vi "S4GUI.vi"(7 "Tab ObsEng":enum32{"Obs", "CCD modes", "Eng"}(tab)) -> ()   [LabVIEW 2018] (continued)
            n3853 = call-dynamic "Write sequencia.vi"("error in (no error)"=w8967, "sequencia"=w8969, "Opt_Selector in"=w8970) -> ("error out"=w8962:errorcluster, "Opt_Selector out"=w8963:refnum<class "Opt_Selector.lvclass">)  [unwired: 7 in]
            n3854 = call-dynamic "Read State Machine.vi"("error in (no error)"=w8962, "Device in"=w8963) -> ("error out"=w8965:errorcluster, "State Machine.lvclass"=w8960:refnum<class "State Machine.lvclass">, "Device out"=w8961:refnum<class "Opt_Selector.lvclass">)  [unwired: 7 in]
            n3855 = call "Next State.vi"("error in (no error)"=w8965, "New_State"=10, "State Machine in"=w8960) -> ("error out"=w8964:errorcluster, "State Machine out"=w8959:refnum<class "State Machine.lvclass">)  [unwired: 7 in]
            n3856 = call-dynamic "Write State Machine.vi"("error in (no error)"=w8964, "State Machine.lvclass"=w8959, "Device in"=w8961) -> ("error out"=w8958:errorcluster, "Device out"=w8957:refnum<class "Opt_Selector.lvclass">)  [unwired: 7 in]
            n3857 = call "Write WPROT.vi"("error in (no error)"=w8958, "Opt_Selector.lvclass"=w8957, "Instrument in"=w8976) -> ("error out"=w8955:errorcluster, "Instrument out"=w8956:refnum<class "Instrument.lvclass">)  [unwired: 7 in]
            n3858 = call "Write Instrument.lvclass.vi"("error in (no error)"=w8955, "Instrument.lvclass"=w8956, "S4ACS_GUI in"=w8974) -> ("error out"=w8977:errorcluster, "S4ACS_GUI out"=w8978:refnum<class "S4GUI.lvclass">)  [unwired: 7 in]
            n3859 = call-dynamic "Write ciclos.vi"("error in (no error)"=w8977, "ciclos"=u32 0, "S4ACS_GUI in"=w8978) -> ("error out"=w8951:errorcluster, "S4ACS_GUI out"=w8952:refnum<class "S4GUI.lvclass">)  [unwired: 7 in]
          }
          frame Enabled {
            w9068 = FALSE ("Wait Until Done")
            n3860 = call <vilib>:"Application Directory.vi"() -> ("Application Directory"=w9063:path)
            n3861 = Build Path(base path=w9063, name or relative path="MsgAbortSync.vi") -> (appended path=w9071:path)
            n3862 = Open VI Reference(vi path=w9071, error in (no error)=w9066) -> (vi reference=w9070:refnum<vi>, error out=w9069:errorcluster)  [unwired: 4 in]
            n3863 = invoke class="VI" method="Run VI"(reference=w9070, error in=w9069, "Wait until done"=w9068, "Auto Dispose Ref"=w9068) -> (error out=w9065:errorcluster)  [unwired: 1 in, 4 out]
          }
        }
        n3864 = property on="#Cycles Done" class="Slide (strict)"(error in=w8947, "Scale.Maximum"=w8949, "Scale.Minimum"=w8949) -> (error out=w8950:errorcluster)  [unwired: 1 in, 1 out]
      }
      event "Pause SM": Value Change {
        n3865 = event-data() -> ()  [unwired: 1 in, 6 out]
        n3866 = call-dynamic "Write User Event.vi"("error in (no error)"=w9075, "User Event"="PAUSE SM CLICKED", "S4GUI in"=w9076) -> ("error out"=w9073:errorcluster, "S4GUI out"=w9074:refnum<class "S4GUI.lvclass">)  [unwired: 7 in]
        n3867 = disable-structure shown="Enabled" {
          disable-tunnel: w9074 -> [w9090 w9100]
          disable-tunnel: w9073 -> [w9089 w9101]
          disable-tunnel: [w9080 w9100] -> w9078
          disable-tunnel: [w9079 w9099] -> w9077
          frame Disabled {
            n3868 = disable-structure shown="Enabled" {
              disable-tunnel: w9090 -> [w9094 w9097]
              disable-tunnel: w9089 -> [w9093 w9096]
              disable-tunnel: [w9092 w9097] -> w9083
              disable-tunnel: [w9091 w9096] -> w9082
              frame Disabled {
                n3869 = call-dynamic "Write paused.vi"("error in (no error)"=w9093, "paused"=TRUE ("stopped"), "S4ACS_GUI in"=w9094) -> ("error out"=w9091:errorcluster, "S4ACS_GUI out"=w9092:refnum<class "S4GUI.lvclass">)  [unwired: 7 in]
              }
              frame Enabled {
              }
            }
            n3870 = call-dynamic "Read Obs_state.vi"("error in (no error)"=w9082, "S4ACS_GUI in"=w9083) -> ("error out"=w9086:errorcluster, "Obs_state"=w9088:u32, "S4ACS_GUI out"=w9087:refnum<class "S4GUI.lvclass">)  [unwired: 7 in]
            n3871 = call-dynamic "Write Obs_prevstate.vi"("error in (no error)"=w9086, "Obs_prevstate"=w9088, "S4ACS_GUI in"=w9087) -> ("error out"=w9084:errorcluster, "S4ACS_GUI out"=w9085:refnum<class "S4GUI.lvclass">)  [unwired: 7 in]
            n3872 = call-dynamic "Write Obs_state.vi"("error in (no error)"=w9084, "Obs_state"=u32 400, "S4ACS_GUI in"=w9085) -> ("error out"=w9079:errorcluster, "S4ACS_GUI out"=w9080:refnum<class "S4GUI.lvclass">)  [unwired: 7 in]
          }
          frame Enabled {
            w9103 = FALSE ("Wait Until Done")
            n3873 = call <vilib>:"Application Directory.vi"() -> ("Application Directory"=w9098:path)
            n3874 = Build Path(base path=w9098, name or relative path="MsgPauseSync.vi") -> (appended path=w9106:path)
            n3875 = Open VI Reference(vi path=w9106, error in (no error)=w9101) -> (vi reference=w9105:refnum<vi>, error out=w9104:errorcluster)  [unwired: 4 in]
            n3876 = invoke class="VI" method="Run VI"(reference=w9105, error in=w9104, "Wait until done"=w9103, "Auto Dispose Ref"=w9103) -> (error out=w9099:errorcluster)  [unwired: 1 in, 4 out]
          }
        }
      }
      event "Abort ch1": Value Change {
        n3877 = event-data() -> ()  [unwired: 1 in, 6 out]
        n3878 = disable-structure shown="Enabled" {
          disable-tunnel: w9110 -> [w9143 w9165]
          disable-tunnel: w9109 -> [w9141 w9159]
          disable-tunnel: [w9123 w9158] -> w9108
          disable-tunnel: [w9111 w9165] -> w9107
          frame Disabled {
            # "Para movimento \nda lamina retardadora"
            # "Restaura a última sequência de lâminas"
            n3879 = call-dynamic "Read AcquisitionA.vi"("error in (no error)"=w9141, "S4ACS_GUI in"=w9143) -> ("error out"=w9146:errorcluster, "Acquisition.lvclass"=w9145:refnum<class "Acquisition.lvclass">, "S4ACS_GUI out"=w9142:refnum<class "S4GUI.lvclass">)  [unwired: 7 in]
            n3880 = call-dynamic "Read Channel.vi"("error in (no error)"=w9146, "Acquisition in"=w9145) -> ("error out"=w9148:errorcluster, "Channel.lvclass"=w9147:refnum<class "Channel.lvclass">, "Acquisition out"=w9154:refnum<class "Acquisition.lvclass">)  [unwired: 7 in]
            n3881 = call-dynamic "Read State Machine.vi"("error in (no error)"=w9148, "Device in"=w9147) -> ("error out"=w9150:errorcluster, "State Machine.lvclass"=w9149:refnum<class "State Machine.lvclass">, "Device out"=w9152:refnum<class "Channel.lvclass">)  [unwired: 7 in]
            n3882 = call "Next State.vi"("error in (no error)"=w9150, "New_State"=u32 80, "State Machine in"=w9149) -> ("error out"=w9153:errorcluster, "State Machine out"=w9151:refnum<class "State Machine.lvclass">)  [unwired: 7 in]
            n3883 = call-dynamic "Write State Machine.vi"("error in (no error)"=w9153, "State Machine.lvclass"=w9151, "Device in"=w9152) -> ("error out"=w9155:errorcluster, "Device out"=w9156:refnum<class "Channel.lvclass">)  [unwired: 7 in]
            n3884 = call-dynamic "Write Channel.vi"("error in (no error)"=w9155, "Channel.lvclass"=w9156, "Acquisition in"=w9154) -> ("error out"=w9138:errorcluster, "Acquisition out"=w9139:refnum<class "Acquisition.lvclass">)  [unwired: 7 in]
            n3885 = call-dynamic "Write Acq_state.vi"("error in (no error)"=w9138, "Acq_state"=u32 0, "Acquisition in"=w9139) -> ("error out"=w9137:errorcluster, "Acquisition out"=w9136:refnum<class "Acquisition.lvclass">)  [unwired: 7 in]
            n3886 = call-dynamic "Write AcquisitionA.vi"("error in (no error)"=w9137, "Acquisition.lvclass"=w9136, "S4ACS_GUI in"=w9142) -> ("error out"=w9124:errorcluster, "S4ACS_GUI out"=w9122:refnum<class "S4GUI.lvclass">)  [unwired: 7 in]
            n3887 = call "Read Instrument.lvclass.vi"("error in (no error)"=w9124, "S4ACS_GUI in"=w9122) -> ("error out"=w9131:errorcluster, "Instrument.lvclass"=w9134:refnum<class "Instrument.lvclass">, "S4ACS_GUI out"=w9135:refnum<class "S4GUI.lvclass">)  [unwired: 7 in]
            n3888 = call "Read WPROT.vi"("error in (no error)"=w9131, "Instrument in"=w9134) -> ("error out"=w9130:errorcluster, "Opt_Selector.lvclass"=w9132:refnum<class "Opt_Selector.lvclass">, "Instrument out"=w9133:refnum<class "Instrument.lvclass">)  [unwired: 7 in]
            n3889 = call-dynamic "Read sequencia_ant.vi"("error in (no error)"=w9130, "Opt_Selector in"=w9132) -> ("error out"=w9126:errorcluster, "sequencia_ant"=w9125:u16, "Opt_Selector out"=w9127:refnum<class "Opt_Selector.lvclass">)  [unwired: 7 in]
            n3890 = call-dynamic "Write sequencia.vi"("error in (no error)"=w9126, "sequencia"=w9125, "Opt_Selector in"=w9127) -> ("error out"=w9115:errorcluster, "Opt_Selector out"=w9116:refnum<class "Opt_Selector.lvclass">)  [unwired: 7 in]
            n3891 = call-dynamic "Read State Machine.vi"("error in (no error)"=w9115, "Device in"=w9116) -> ("error out"=w9118:errorcluster, "State Machine.lvclass"=w9121:refnum<class "State Machine.lvclass">, "Device out"=w9114:refnum<class "Opt_Selector.lvclass">)  [unwired: 7 in]
            n3892 = call "Next State.vi"("error in (no error)"=w9118, "New_State"=10, "State Machine in"=w9121) -> ("error out"=w9117:errorcluster, "State Machine out"=w9120:refnum<class "State Machine.lvclass">)  [unwired: 7 in]
            n3893 = call-dynamic "Write State Machine.vi"("error in (no error)"=w9117, "State Machine.lvclass"=w9120, "Device in"=w9114) -> ("error out"=w9112:errorcluster, "Device out"=w9113:refnum<class "Opt_Selector.lvclass">)  [unwired: 7 in]
            n3894 = call "Write WPROT.vi"("error in (no error)"=w9112, "Opt_Selector.lvclass"=w9113, "Instrument in"=w9133) -> ("error out"=w9129:errorcluster, "Instrument out"=w9128:refnum<class "Instrument.lvclass">)  [unwired: 7 in]
            n3895 = call "Write Instrument.lvclass.vi"("error in (no error)"=w9129, "Instrument.lvclass"=w9128, "S4ACS_GUI in"=w9135) -> ("error out"=w9123:errorcluster, "S4ACS_GUI out"=w9111:refnum<class "S4GUI.lvclass">)  [unwired: 7 in]
          }
          frame Enabled {
            w9161 = FALSE ("Wait Until Done")
            n3896 = call <vilib>:"Application Directory.vi"() -> ("Application Directory"=w9157:path)
            n3897 = Build Path(base path=w9157, name or relative path="MsgAbort1.vi") -> (appended path=w9164:path)
            n3898 = Open VI Reference(vi path=w9164, error in (no error)=w9159) -> (vi reference=w9163:refnum<vi>, error out=w9162:errorcluster)  [unwired: 4 in]
            n3899 = invoke class="VI" method="Run VI"(reference=w9163, error in=w9162, "Wait until done"=w9161, "Auto Dispose Ref"=w9161) -> (error out=w9158:errorcluster)  [unwired: 1 in, 4 out]
          }
        }
      }
      event "Abort ch2": Value Change {
        n3900 = event-data() -> ()  [unwired: 1 in, 6 out]
        n3901 = disable-structure shown="Enabled" {
          disable-tunnel: w9169 -> [w9202 w9218]
          disable-tunnel: w9168 -> [w9200 w9219]
          disable-tunnel: [w9182 w9217] -> w9167
          disable-tunnel: [w9170 w9218] -> w9166
          frame Disabled {
            # "Para movimento \nda lamina retardadora"
            # "Restaura a última sequência de lâminas"
            n3902 = call "Read AcquisitionB.vi"("error in (no error)"=w9200, "S4ACS_GUI in"=w9202) -> ("error out"=w9205:errorcluster, "Acquisition.lvclass"=w9204:refnum<class "Acquisition.lvclass">, "S4ACS_GUI out"=w9201:refnum<class "S4GUI.lvclass">)  [unwired: 7 in]
            n3903 = call-dynamic "Read Channel.vi"("error in (no error)"=w9205, "Acquisition in"=w9204) -> ("error out"=w9207:errorcluster, "Channel.lvclass"=w9206:refnum<class "Channel.lvclass">, "Acquisition out"=w9213:refnum<class "Acquisition.lvclass">)  [unwired: 7 in]
            n3904 = call-dynamic "Read State Machine.vi"("error in (no error)"=w9207, "Device in"=w9206) -> ("error out"=w9209:errorcluster, "State Machine.lvclass"=w9208:refnum<class "State Machine.lvclass">, "Device out"=w9211:refnum<class "Channel.lvclass">)  [unwired: 7 in]
            n3905 = call "Next State.vi"("error in (no error)"=w9209, "New_State"=u32 80, "State Machine in"=w9208) -> ("error out"=w9212:errorcluster, "State Machine out"=w9210:refnum<class "State Machine.lvclass">)  [unwired: 7 in]
            n3906 = call-dynamic "Write State Machine.vi"("error in (no error)"=w9212, "State Machine.lvclass"=w9210, "Device in"=w9211) -> ("error out"=w9214:errorcluster, "Device out"=w9215:refnum<class "Channel.lvclass">)  [unwired: 7 in]
            n3907 = call-dynamic "Write Channel.vi"("error in (no error)"=w9214, "Channel.lvclass"=w9215, "Acquisition in"=w9213) -> ("error out"=w9197:errorcluster, "Acquisition out"=w9198:refnum<class "Acquisition.lvclass">)  [unwired: 7 in]
            n3908 = call-dynamic "Write Acq_state.vi"("error in (no error)"=w9197, "Acq_state"=u32 0, "Acquisition in"=w9198) -> ("error out"=w9196:errorcluster, "Acquisition out"=w9195:refnum<class "Acquisition.lvclass">)  [unwired: 7 in]
            n3909 = call "Write AcquisitionB.vi"("error in (no error)"=w9196, "Acquisition.lvclass"=w9195, "S4ACS_GUI in"=w9201) -> ("error out"=w9183:errorcluster, "S4ACS_GUI out"=w9181:refnum<class "S4GUI.lvclass">)  [unwired: 7 in]
            n3910 = call "Read Instrument.lvclass.vi"("error in (no error)"=w9183, "S4ACS_GUI in"=w9181) -> ("error out"=w9190:errorcluster, "Instrument.lvclass"=w9193:refnum<class "Instrument.lvclass">, "S4ACS_GUI out"=w9194:refnum<class "S4GUI.lvclass">)  [unwired: 7 in]
            n3911 = call "Read WPROT.vi"("error in (no error)"=w9190, "Instrument in"=w9193) -> ("error out"=w9189:errorcluster, "Opt_Selector.lvclass"=w9191:refnum<class "Opt_Selector.lvclass">, "Instrument out"=w9192:refnum<class "Instrument.lvclass">)  [unwired: 7 in]
            n3912 = call-dynamic "Read sequencia_ant.vi"("error in (no error)"=w9189, "Opt_Selector in"=w9191) -> ("error out"=w9185:errorcluster, "sequencia_ant"=w9184:u16, "Opt_Selector out"=w9186:refnum<class "Opt_Selector.lvclass">)  [unwired: 7 in]
            n3913 = call-dynamic "Write sequencia.vi"("error in (no error)"=w9185, "sequencia"=w9184, "Opt_Selector in"=w9186) -> ("error out"=w9174:errorcluster, "Opt_Selector out"=w9175:refnum<class "Opt_Selector.lvclass">)  [unwired: 7 in]
            n3914 = call-dynamic "Read State Machine.vi"("error in (no error)"=w9174, "Device in"=w9175) -> ("error out"=w9177:errorcluster, "State Machine.lvclass"=w9180:refnum<class "State Machine.lvclass">, "Device out"=w9173:refnum<class "Opt_Selector.lvclass">)  [unwired: 7 in]
            n3915 = call "Next State.vi"("error in (no error)"=w9177, "New_State"=10, "State Machine in"=w9180) -> ("error out"=w9176:errorcluster, "State Machine out"=w9179:refnum<class "State Machine.lvclass">)  [unwired: 7 in]
            n3916 = call-dynamic "Write State Machine.vi"("error in (no error)"=w9176, "State Machine.lvclass"=w9179, "Device in"=w9173) -> ("error out"=w9171:errorcluster, "Device out"=w9172:refnum<class "Opt_Selector.lvclass">)  [unwired: 7 in]
            n3917 = call "Write WPROT.vi"("error in (no error)"=w9171, "Opt_Selector.lvclass"=w9172, "Instrument in"=w9192) -> ("error out"=w9188:errorcluster, "Instrument out"=w9187:refnum<class "Instrument.lvclass">)  [unwired: 7 in]
            n3918 = call "Write Instrument.lvclass.vi"("error in (no error)"=w9188, "Instrument.lvclass"=w9187, "S4ACS_GUI in"=w9194) -> ("error out"=w9182:errorcluster, "S4ACS_GUI out"=w9170:refnum<class "S4GUI.lvclass">)  [unwired: 7 in]
          }
          frame Enabled {
            w9221 = FALSE ("Wait Until Done")
            n3919 = call <vilib>:"Application Directory.vi"() -> ("Application Directory"=w9216:path)
            n3920 = Build Path(base path=w9216, name or relative path="MsgAbort2.vi") -> (appended path=w9224:path)
            n3921 = Open VI Reference(vi path=w9224, error in (no error)=w9219) -> (vi reference=w9223:refnum<vi>, error out=w9222:errorcluster)  [unwired: 4 in]
            n3922 = invoke class="VI" method="Run VI"(reference=w9223, error in=w9222, "Wait until done"=w9221, "Auto Dispose Ref"=w9221) -> (error out=w9217:errorcluster)  [unwired: 1 in, 4 out]
          }
        }
      }
      event "Abort ch3": Value Change {
        n3923 = event-data() -> ()  [unwired: 1 in, 6 out]
        n3924 = disable-structure shown="Enabled" {
          disable-tunnel: w9228 -> [w9261 w9277]
          disable-tunnel: w9227 -> [w9259 w9278]
          disable-tunnel: [w9241 w9276] -> w9226
          disable-tunnel: [w9229 w9277] -> w9225
          frame Disabled {
            # "Para movimento \nda lamina retardadora"
            # "Restaura a última sequência de lâminas"
            n3925 = call-dynamic "Read AcquisitionC.vi"("error in (no error)"=w9259, "S4ACS_GUI in"=w9261) -> ("error out"=w9264:errorcluster, "Acquisition.lvclass"=w9263:refnum<class "Acquisition.lvclass">, "S4ACS_GUI out"=w9260:refnum<class "S4GUI.lvclass">)  [unwired: 7 in]
            n3926 = call-dynamic "Read Channel.vi"("error in (no error)"=w9264, "Acquisition in"=w9263) -> ("error out"=w9266:errorcluster, "Channel.lvclass"=w9265:refnum<class "Channel.lvclass">, "Acquisition out"=w9272:refnum<class "Acquisition.lvclass">)  [unwired: 7 in]
            n3927 = call-dynamic "Read State Machine.vi"("error in (no error)"=w9266, "Device in"=w9265) -> ("error out"=w9268:errorcluster, "State Machine.lvclass"=w9267:refnum<class "State Machine.lvclass">, "Device out"=w9270:refnum<class "Channel.lvclass">)  [unwired: 7 in]
            n3928 = call "Next State.vi"("error in (no error)"=w9268, "New_State"=u32 80, "State Machine in"=w9267) -> ("error out"=w9271:errorcluster, "State Machine out"=w9269:refnum<class "State Machine.lvclass">)  [unwired: 7 in]
            n3929 = call-dynamic "Write State Machine.vi"("error in (no error)"=w9271, "State Machine.lvclass"=w9269, "Device in"=w9270) -> ("error out"=w9273:errorcluster, "Device out"=w9274:refnum<class "Channel.lvclass">)  [unwired: 7 in]
            n3930 = call-dynamic "Write Channel.vi"("error in (no error)"=w9273, "Channel.lvclass"=w9274, "Acquisition in"=w9272) -> ("error out"=w9256:errorcluster, "Acquisition out"=w9257:refnum<class "Acquisition.lvclass">)  [unwired: 7 in]
            n3931 = call-dynamic "Write Acq_state.vi"("error in (no error)"=w9256, "Acq_state"=u32 0, "Acquisition in"=w9257) -> ("error out"=w9255:errorcluster, "Acquisition out"=w9254:refnum<class "Acquisition.lvclass">)  [unwired: 7 in]
            n3932 = call-dynamic "Write AcquisitionC.vi"("error in (no error)"=w9255, "Acquisition.lvclass"=w9254, "S4ACS_GUI in"=w9260) -> ("error out"=w9242:errorcluster, "S4ACS_GUI out"=w9240:refnum<class "S4GUI.lvclass">)  [unwired: 7 in]
            n3933 = call "Read Instrument.lvclass.vi"("error in (no error)"=w9242, "S4ACS_GUI in"=w9240) -> ("error out"=w9249:errorcluster, "Instrument.lvclass"=w9252:refnum<class "Instrument.lvclass">, "S4ACS_GUI out"=w9253:refnum<class "S4GUI.lvclass">)  [unwired: 7 in]
            n3934 = call "Read WPROT.vi"("error in (no error)"=w9249, "Instrument in"=w9252) -> ("error out"=w9248:errorcluster, "Opt_Selector.lvclass"=w9250:refnum<class "Opt_Selector.lvclass">, "Instrument out"=w9251:refnum<class "Instrument.lvclass">)  [unwired: 7 in]
            n3935 = call-dynamic "Read sequencia_ant.vi"("error in (no error)"=w9248, "Opt_Selector in"=w9250) -> ("error out"=w9244:errorcluster, "sequencia_ant"=w9243:u16, "Opt_Selector out"=w9245:refnum<class "Opt_Selector.lvclass">)  [unwired: 7 in]
            n3936 = call-dynamic "Write sequencia.vi"("error in (no error)"=w9244, "sequencia"=w9243, "Opt_Selector in"=w9245) -> ("error out"=w9233:errorcluster, "Opt_Selector out"=w9234:refnum<class "Opt_Selector.lvclass">)  [unwired: 7 in]
            n3937 = call-dynamic "Read State Machine.vi"("error in (no error)"=w9233, "Device in"=w9234) -> ("error out"=w9236:errorcluster, "State Machine.lvclass"=w9239:refnum<class "State Machine.lvclass">, "Device out"=w9232:refnum<class "Opt_Selector.lvclass">)  [unwired: 7 in]
            n3938 = call "Next State.vi"("error in (no error)"=w9236, "New_State"=10, "State Machine in"=w9239) -> ("error out"=w9235:errorcluster, "State Machine out"=w9238:refnum<class "State Machine.lvclass">)  [unwired: 7 in]
            n3939 = call-dynamic "Write State Machine.vi"("error in (no error)"=w9235, "State Machine.lvclass"=w9238, "Device in"=w9232) -> ("error out"=w9230:errorcluster, "Device out"=w9231:refnum<class "Opt_Selector.lvclass">)  [unwired: 7 in]
            n3940 = call "Write WPROT.vi"("error in (no error)"=w9230, "Opt_Selector.lvclass"=w9231, "Instrument in"=w9251) -> ("error out"=w9247:errorcluster, "Instrument out"=w9246:refnum<class "Instrument.lvclass">)  [unwired: 7 in]
            n3941 = call "Write Instrument.lvclass.vi"("error in (no error)"=w9247, "Instrument.lvclass"=w9246, "S4ACS_GUI in"=w9253) -> ("error out"=w9241:errorcluster, "S4ACS_GUI out"=w9229:refnum<class "S4GUI.lvclass">)  [unwired: 7 in]
          }
          frame Enabled {
            w9280 = FALSE ("Wait Until Done")
            n3942 = call <vilib>:"Application Directory.vi"() -> ("Application Directory"=w9275:path)
            n3943 = Build Path(base path=w9275, name or relative path="MsgAbort3.vi") -> (appended path=w9283:path)
            n3944 = Open VI Reference(vi path=w9283, error in (no error)=w9278) -> (vi reference=w9282:refnum<vi>, error out=w9281:errorcluster)  [unwired: 4 in]
            n3945 = invoke class="VI" method="Run VI"(reference=w9282, error in=w9281, "Wait until done"=w9280, "Auto Dispose Ref"=w9280) -> (error out=w9276:errorcluster)  [unwired: 1 in, 4 out]
          }
        }
      }
      event "Abort ch4": Value Change {
        n3946 = event-data() -> ()  [unwired: 1 in, 6 out]
        n3947 = disable-structure shown="Enabled" {
          disable-tunnel: w9287 -> [w9320 w9336]
          disable-tunnel: w9286 -> [w9318 w9337]
          disable-tunnel: [w9300 w9335] -> w9285
          disable-tunnel: [w9288 w9336] -> w9284
          frame Disabled {
            # "Para movimento \nda lamina retardadora"
            # "Restaura a última sequência de lâminas"
            n3948 = call-dynamic "Read AcquisitionD.vi"("error in (no error)"=w9318, "S4ACS_GUI in"=w9320) -> ("error out"=w9323:errorcluster, "Acquisition.lvclass"=w9322:refnum<class "Acquisition.lvclass">, "S4ACS_GUI out"=w9319:refnum<class "S4GUI.lvclass">)  [unwired: 7 in]
            n3949 = call-dynamic "Read Channel.vi"("error in (no error)"=w9323, "Acquisition in"=w9322) -> ("error out"=w9325:errorcluster, "Channel.lvclass"=w9324:refnum<class "Channel.lvclass">, "Acquisition out"=w9331:refnum<class "Acquisition.lvclass">)  [unwired: 7 in]
            n3950 = call-dynamic "Read State Machine.vi"("error in (no error)"=w9325, "Device in"=w9324) -> ("error out"=w9327:errorcluster, "State Machine.lvclass"=w9326:refnum<class "State Machine.lvclass">, "Device out"=w9329:refnum<class "Channel.lvclass">)  [unwired: 7 in]
            n3951 = call "Next State.vi"("error in (no error)"=w9327, "New_State"=u32 80, "State Machine in"=w9326) -> ("error out"=w9330:errorcluster, "State Machine out"=w9328:refnum<class "State Machine.lvclass">)  [unwired: 7 in]
            n3952 = call-dynamic "Write State Machine.vi"("error in (no error)"=w9330, "State Machine.lvclass"=w9328, "Device in"=w9329) -> ("error out"=w9332:errorcluster, "Device out"=w9333:refnum<class "Channel.lvclass">)  [unwired: 7 in]
            n3953 = call-dynamic "Write Channel.vi"("error in (no error)"=w9332, "Channel.lvclass"=w9333, "Acquisition in"=w9331) -> ("error out"=w9315:errorcluster, "Acquisition out"=w9316:refnum<class "Acquisition.lvclass">)  [unwired: 7 in]
            n3954 = call-dynamic "Write Acq_state.vi"("error in (no error)"=w9315, "Acq_state"=u32 0, "Acquisition in"=w9316) -> ("error out"=w9314:errorcluster, "Acquisition out"=w9313:refnum<class "Acquisition.lvclass">)  [unwired: 7 in]
            n3955 = call-dynamic "Write AcquisitionD.vi"("error in (no error)"=w9314, "Acquisition.lvclass"=w9313, "S4ACS_GUI in"=w9319) -> ("error out"=w9301:errorcluster, "S4ACS_GUI out"=w9299:refnum<class "S4GUI.lvclass">)  [unwired: 7 in]
            n3956 = call "Read Instrument.lvclass.vi"("error in (no error)"=w9301, "S4ACS_GUI in"=w9299) -> ("error out"=w9308:errorcluster, "Instrument.lvclass"=w9311:refnum<class "Instrument.lvclass">, "S4ACS_GUI out"=w9312:refnum<class "S4GUI.lvclass">)  [unwired: 7 in]
            n3957 = call "Read WPROT.vi"("error in (no error)"=w9308, "Instrument in"=w9311) -> ("error out"=w9307:errorcluster, "Opt_Selector.lvclass"=w9309:refnum<class "Opt_Selector.lvclass">, "Instrument out"=w9310:refnum<class "Instrument.lvclass">)  [unwired: 7 in]
            n3958 = call-dynamic "Read sequencia_ant.vi"("error in (no error)"=w9307, "Opt_Selector in"=w9309) -> ("error out"=w9303:errorcluster, "sequencia_ant"=w9302:u16, "Opt_Selector out"=w9304:refnum<class "Opt_Selector.lvclass">)  [unwired: 7 in]
            n3959 = call-dynamic "Write sequencia.vi"("error in (no error)"=w9303, "sequencia"=w9302, "Opt_Selector in"=w9304) -> ("error out"=w9292:errorcluster, "Opt_Selector out"=w9293:refnum<class "Opt_Selector.lvclass">)  [unwired: 7 in]
            n3960 = call-dynamic "Read State Machine.vi"("error in (no error)"=w9292, "Device in"=w9293) -> ("error out"=w9295:errorcluster, "State Machine.lvclass"=w9298:refnum<class "State Machine.lvclass">, "Device out"=w9291:refnum<class "Opt_Selector.lvclass">)  [unwired: 7 in]
            n3961 = call "Next State.vi"("error in (no error)"=w9295, "New_State"=10, "State Machine in"=w9298) -> ("error out"=w9294:errorcluster, "State Machine out"=w9297:refnum<class "State Machine.lvclass">)  [unwired: 7 in]
            n3962 = call-dynamic "Write State Machine.vi"("error in (no error)"=w9294, "State Machine.lvclass"=w9297, "Device in"=w9291) -> ("error out"=w9289:errorcluster, "Device out"=w9290:refnum<class "Opt_Selector.lvclass">)  [unwired: 7 in]
            n3963 = call "Write WPROT.vi"("error in (no error)"=w9289, "Opt_Selector.lvclass"=w9290, "Instrument in"=w9310) -> ("error out"=w9306:errorcluster, "Instrument out"=w9305:refnum<class "Instrument.lvclass">)  [unwired: 7 in]
            n3964 = call "Write Instrument.lvclass.vi"("error in (no error)"=w9306, "Instrument.lvclass"=w9305, "S4ACS_GUI in"=w9312) -> ("error out"=w9300:errorcluster, "S4ACS_GUI out"=w9288:refnum<class "S4GUI.lvclass">)  [unwired: 7 in]
          }
          frame Enabled {
            w9339 = FALSE ("Wait Until Done")
            n3965 = call <vilib>:"Application Directory.vi"() -> ("Application Directory"=w9334:path)
            n3966 = Build Path(base path=w9334, name or relative path="MsgAbort4.vi") -> (appended path=w9342:path)
            n3967 = Open VI Reference(vi path=w9342, error in (no error)=w9337) -> (vi reference=w9341:refnum<vi>, error out=w9340:errorcluster)  [unwired: 4 in]
            n3968 = invoke class="VI" method="Run VI"(reference=w9341, error in=w9340, "Wait until done"=w9339, "Auto Dispose Ref"=w9339) -> (error out=w9335:errorcluster)  [unwired: 1 in, 4 out]
          }
        }
      }
      event "SyncBox": Value Change {
        n3969 = event-data() -> ()  [unwired: 1 in, 4 out]
        n3970 = call-dynamic "Read Sync Box.lvclass.vi"("error in (no error)"=w9345, "SPARC4_AC in"=w9346) -> ("error out"=w9361:errorcluster, "Sync Box.lvclass"=w9362:refnum<class "Sync Box.lvclass">, "SPARC4_AC out"=w9350:refnum<class "S4GUI.lvclass">)  [unwired: 7 in]
        n3971 = call-dynamic "Read Trigger.lvclass.vi"("error in (no error)"=w9361, "Sync Box in"=w9362) -> ("error out"=w9359:errorcluster, "Trigger.lvclass"=w9360:refnum<class "Trigger.lvclass">, "Sync Box out"=w9353:refnum<class "Sync Box.lvclass">)  [unwired: 7 in]
        n3972 = call-dynamic "Read State Machine.vi"("error in (no error)"=w9359, "Device in"=w9360) -> ("error out"=w9357:errorcluster, "State Machine.lvclass"=w9358:refnum<class "State Machine.lvclass">, "Device out"=w9354:refnum<class "Trigger.lvclass">)  [unwired: 7 in]
        n3973 = call "Next State.vi"("error in (no error)"=w9357, "New_State"=u32 1, "State Machine in"=w9358) -> ("error out"=w9352:errorcluster, "State Machine out"=w9355:refnum<class "State Machine.lvclass">)  [unwired: 7 in]
        n3974 = call-dynamic "Write State Machine.vi"("error in (no error)"=w9352, "State Machine.lvclass"=w9355, "Device in"=w9354) -> ("error out"=w9348:errorcluster, "Device out"=w9347:refnum<class "Trigger.lvclass">)  [unwired: 7 in]
        n3975 = call-dynamic "Write Trigger.lvclass.vi"("error in (no error)"=w9348, "Trigger.lvclass"=w9347, "Sync Box in"=w9353) -> ("error out"=w9349:errorcluster, "Sync Box out"=w9351:refnum<class "Sync Box.lvclass">)  [unwired: 7 in]
        n3976 = call-dynamic "Write Sync Box.lvclass.vi"("error in (no error)"=w9349, "Sync Box.lvclass"=w9351, "SPARC4_AC in"=w9350) -> ("error out"=w9344:errorcluster, "SPARC4_AC out"=w9343:refnum<class "S4GUI.lvclass">)  [unwired: 7 in]
      }
      event "Fire manual", "Fire": Value Change {
        n3977 = event-data() -> ()  [unwired: 1 in, 4 out]
        n3978 = call-dynamic "Read Sync Box.lvclass.vi"("error in (no error)"=w9365, "SPARC4_AC in"=w9366) -> ("error out"=w9381:errorcluster, "Sync Box.lvclass"=w9382:refnum<class "Sync Box.lvclass">, "SPARC4_AC out"=w9370:refnum<class "S4GUI.lvclass">)  [unwired: 7 in]
        n3979 = call-dynamic "Read Trigger.lvclass.vi"("error in (no error)"=w9381, "Sync Box in"=w9382) -> ("error out"=w9379:errorcluster, "Trigger.lvclass"=w9380:refnum<class "Trigger.lvclass">, "Sync Box out"=w9373:refnum<class "Sync Box.lvclass">)  [unwired: 7 in]
        n3980 = call-dynamic "Read State Machine.vi"("error in (no error)"=w9379, "Device in"=w9380) -> ("error out"=w9377:errorcluster, "State Machine.lvclass"=w9378:refnum<class "State Machine.lvclass">, "Device out"=w9374:refnum<class "Trigger.lvclass">)  [unwired: 7 in]
        n3981 = call "Next State.vi"("error in (no error)"=w9377, "New_State"=u32 40, "State Machine in"=w9378) -> ("error out"=w9372:errorcluster, "State Machine out"=w9375:refnum<class "State Machine.lvclass">)  [unwired: 7 in]
        n3982 = call-dynamic "Write State Machine.vi"("error in (no error)"=w9372, "State Machine.lvclass"=w9375, "Device in"=w9374) -> ("error out"=w9368:errorcluster, "Device out"=w9367:refnum<class "Trigger.lvclass">)  [unwired: 7 in]
        n3983 = call-dynamic "Write Trigger.lvclass.vi"("error in (no error)"=w9368, "Trigger.lvclass"=w9367, "Sync Box in"=w9373) -> ("error out"=w9369:errorcluster, "Sync Box out"=w9371:refnum<class "Sync Box.lvclass">)  [unwired: 7 in]
        n3984 = call-dynamic "Write Sync Box.lvclass.vi"("error in (no error)"=w9369, "Sync Box.lvclass"=w9371, "SPARC4_AC in"=w9370) -> ("error out"=w9364:errorcluster, "SPARC4_AC out"=w9363:refnum<class "S4GUI.lvclass">)  [unwired: 7 in]
      }
      event "Select Trigger Mode": Value Change {
        n3985 = event-data() -> ("NewVal"=w9384:bool)  [unwired: 1 in, 2 out]
        n3986 = call-dynamic "Read Sync Box.lvclass.vi"("error in (no error)"=w9392, "SPARC4_AC in"=w9393) -> ("error out"=w9404:errorcluster, "Sync Box.lvclass"=w9405:refnum<class "Sync Box.lvclass">, "SPARC4_AC out"=w9397:refnum<class "S4GUI.lvclass">)  [unwired: 7 in]
        n3987 = call-dynamic "Read Trigger.lvclass.vi"("error in (no error)"=w9404, "Sync Box in"=w9405) -> ("error out"=w9385:errorcluster, "Trigger.lvclass"=w9388:refnum<class "Trigger.lvclass">, "Sync Box out"=w9400:refnum<class "Sync Box.lvclass">)  [unwired: 7 in]
        n3988 = call-dynamic "Write Trigger Mode Target.vi"("error in (no error)"=w9385, "Trigger Mode Target"=w9384, "Trigger in"=w9388) -> ("error out"=w9386:errorcluster, "Trigger out"=w9387:refnum<class "Trigger.lvclass">)  [unwired: 7 in]
        n3989 = call-dynamic "Read State Machine.vi"("error in (no error)"=w9386, "Device in"=w9387) -> ("error out"=w9389:errorcluster, "State Machine.lvclass"=w9390:refnum<class "State Machine.lvclass">, "Device out"=w9401:refnum<class "Trigger.lvclass">)  [unwired: 7 in]
        n3990 = call "Next State.vi"("error in (no error)"=w9389, "New_State"=u32 30, "State Machine in"=w9390) -> ("error out"=w9399:errorcluster, "State Machine out"=w9402:refnum<class "State Machine.lvclass">)  [unwired: 7 in]
        n3991 = call-dynamic "Write State Machine.vi"("error in (no error)"=w9399, "State Machine.lvclass"=w9402, "Device in"=w9401) -> ("error out"=w9395:errorcluster, "Device out"=w9394:refnum<class "Trigger.lvclass">)  [unwired: 7 in]
        n3992 = call-dynamic "Write Trigger.lvclass.vi"("error in (no error)"=w9395, "Trigger.lvclass"=w9394, "Sync Box in"=w9400) -> ("error out"=w9396:errorcluster, "Sync Box out"=w9398:refnum<class "Sync Box.lvclass">)  [unwired: 7 in]
        n3993 = call-dynamic "Write Sync Box.lvclass.vi"("error in (no error)"=w9396, "Sync Box.lvclass"=w9398, "SPARC4_AC in"=w9397) -> ("error out"=w9391:errorcluster, "SPARC4_AC out"=w9383:refnum<class "S4GUI.lvclass">)  [unwired: 7 in]
      }
      event "Set SyncBox": Value Change {
        n3994 = event-data() -> ()  [unwired: 1 in, 4 out]
        n3995 = call-dynamic "Read Sync Box.lvclass.vi"("error in (no error)"=w9408, "SPARC4_AC in"=w9409) -> ("error out"=w9424:errorcluster, "Sync Box.lvclass"=w9425:refnum<class "Sync Box.lvclass">, "SPARC4_AC out"=w9413:refnum<class "S4GUI.lvclass">)  [unwired: 7 in]
        n3996 = call-dynamic "Read Trigger.lvclass.vi"("error in (no error)"=w9424, "Sync Box in"=w9425) -> ("error out"=w9422:errorcluster, "Trigger.lvclass"=w9423:refnum<class "Trigger.lvclass">, "Sync Box out"=w9416:refnum<class "Sync Box.lvclass">)  [unwired: 7 in]
        n3997 = call-dynamic "Read State Machine.vi"("error in (no error)"=w9422, "Device in"=w9423) -> ("error out"=w9420:errorcluster, "State Machine.lvclass"=w9421:refnum<class "State Machine.lvclass">, "Device out"=w9417:refnum<class "Trigger.lvclass">)  [unwired: 7 in]
        n3998 = call "Next State.vi"("error in (no error)"=w9420, "New_State"=u32 10, "State Machine in"=w9421) -> ("error out"=w9415:errorcluster, "State Machine out"=w9418:refnum<class "State Machine.lvclass">)  [unwired: 7 in]
        n3999 = call-dynamic "Write State Machine.vi"("error in (no error)"=w9415, "State Machine.lvclass"=w9418, "Device in"=w9417) -> ("error out"=w9411:errorcluster, "Device out"=w9410:refnum<class "Trigger.lvclass">)  [unwired: 7 in]
        n4000 = call-dynamic "Write Trigger.lvclass.vi"("error in (no error)"=w9411, "Trigger.lvclass"=w9410, "Sync Box in"=w9416) -> ("error out"=w9412:errorcluster, "Sync Box out"=w9414:refnum<class "Sync Box.lvclass">)  [unwired: 7 in]
        n4001 = call-dynamic "Write Sync Box.lvclass.vi"("error in (no error)"=w9412, "Sync Box.lvclass"=w9414, "SPARC4_AC in"=w9413) -> ("error out"=w9407:errorcluster, "SPARC4_AC out"=w9406:refnum<class "S4GUI.lvclass">)  [unwired: 7 in]
      }
      event "Set Focus": Value Change {
        n4002 = event-data() -> ("NewVal"=w9426:bool)  [unwired: 1 in]
        n4003 = case shown="True" w9426 {
          tunnel: w9430 -> [w9432 w9441]
          tunnel: w9429 -> [w9431 w9440]
          tunnel: [w9431 w9439] -> w9428
          tunnel: [w9432 w9438] -> w9427
          frame False {
          }
          frame True {
            n4004 = call-dynamic "Read TelFocus.lvclass.vi"("error in (no error)"=w9440, "S4GUI in"=w9441) -> ("error out"=w9454:errorcluster, "TelFocus.lvclass"=w9455:refnum<class "TelFocus.lvclass">, "S4GUI out"=w9445:refnum<class "S4GUI.lvclass">)  [unwired: 7 in]
            n4005 = call-dynamic "Read SecMirror.lvclass.vi"("error in (no error)"=w9454, "TelFocus in"=w9455) -> ("error out"=w9434:errorcluster, "SecMirror.lvclass"=w9437:refnum<class "SecMirror.lvclass">, "TelFocus out"=w9448:refnum<class "TelFocus.lvclass">)  [unwired: 7 in]
            n4006 = call-dynamic "Write target.vi"("error in (no error)"=w9434, "target"="Target focus", "SecMirror in"=w9437) -> ("error out"=w9433:errorcluster, "SecMirror out"=w9436:refnum<class "SecMirror.lvclass">)  [unwired: 7 in]
            n4007 = call-dynamic "Read State Machine.vi"("error in (no error)"=w9433, "Device in"=w9436) -> ("error out"=w9452:errorcluster, "State Machine.lvclass"=w9453:refnum<class "State Machine.lvclass">, "Device out"=w9449:refnum<class "SecMirror.lvclass">)  [unwired: 7 in]
            n4008 = call "Next State.vi"("error in (no error)"=w9452, "New_State"=1, "State Machine in"=w9453) -> ("error out"=w9447:errorcluster, "State Machine out"=w9450:refnum<class "State Machine.lvclass">)  [unwired: 7 in]
            n4009 = call-dynamic "Write State Machine.vi"("error in (no error)"=w9447, "State Machine.lvclass"=w9450, "Device in"=w9449) -> ("error out"=w9443:errorcluster, "Device out"=w9442:refnum<class "SecMirror.lvclass">)  [unwired: 7 in]
            n4010 = call-dynamic "Write SecMirror.lvclass.vi"("error in (no error)"=w9443, "SecMirror.lvclass"=w9442, "TelFocus in"=w9448) -> ("error out"=w9444:errorcluster, "TelFocus out"=w9446:refnum<class "TelFocus.lvclass">)  [unwired: 7 in]
            n4011 = call-dynamic "Write TelFocus.lvclass.vi"("error in (no error)"=w9444, "TelFocus.lvclass"=w9446, "S4GUI in"=w9445) -> ("error out"=w9439:errorcluster, "S4GUI out"=w9438:refnum<class "S4GUI.lvclass">)  [unwired: 7 in]
          }
        }
      }
      event "Set Focus 2": Value Change {
        n4012 = event-data() -> ("NewVal"=w9456:bool)  [unwired: 1 in]
        n4013 = case shown="True" w9456 {
          tunnel: w9460 -> [w9462 w9471]
          tunnel: w9459 -> [w9461 w9470]
          tunnel: [w9461 w9469] -> w9458
          tunnel: [w9462 w9468] -> w9457
          frame False {
          }
          frame True {
            n4014 = call-dynamic "Read TelFocus.lvclass.vi"("error in (no error)"=w9470, "S4GUI in"=w9471) -> ("error out"=w9484:errorcluster, "TelFocus.lvclass"=w9485:refnum<class "TelFocus.lvclass">, "S4GUI out"=w9475:refnum<class "S4GUI.lvclass">)  [unwired: 7 in]
            n4015 = call-dynamic "Read SecMirror.lvclass.vi"("error in (no error)"=w9484, "TelFocus in"=w9485) -> ("error out"=w9465:errorcluster, "SecMirror.lvclass"=w9467:refnum<class "SecMirror.lvclass">, "TelFocus out"=w9478:refnum<class "TelFocus.lvclass">)  [unwired: 7 in]
            n4016 = call-dynamic "Write target.vi"("error in (no error)"=w9465, "target"="Target focus 2", "SecMirror in"=w9467) -> ("error out"=w9464:errorcluster, "SecMirror out"=w9466:refnum<class "SecMirror.lvclass">)  [unwired: 7 in]
            n4017 = call-dynamic "Read State Machine.vi"("error in (no error)"=w9464, "Device in"=w9466) -> ("error out"=w9482:errorcluster, "State Machine.lvclass"=w9483:refnum<class "State Machine.lvclass">, "Device out"=w9479:refnum<class "SecMirror.lvclass">)  [unwired: 7 in]
            n4018 = call "Next State.vi"("error in (no error)"=w9482, "New_State"=1, "State Machine in"=w9483) -> ("error out"=w9477:errorcluster, "State Machine out"=w9480:refnum<class "State Machine.lvclass">)  [unwired: 7 in]
            n4019 = call-dynamic "Write State Machine.vi"("error in (no error)"=w9477, "State Machine.lvclass"=w9480, "Device in"=w9479) -> ("error out"=w9473:errorcluster, "Device out"=w9472:refnum<class "SecMirror.lvclass">)  [unwired: 7 in]
            n4020 = call-dynamic "Write SecMirror.lvclass.vi"("error in (no error)"=w9473, "SecMirror.lvclass"=w9472, "TelFocus in"=w9478) -> ("error out"=w9474:errorcluster, "TelFocus out"=w9476:refnum<class "TelFocus.lvclass">)  [unwired: 7 in]
            n4021 = call-dynamic "Write TelFocus.lvclass.vi"("error in (no error)"=w9474, "TelFocus.lvclass"=w9476, "S4GUI in"=w9475) -> ("error out"=w9469:errorcluster, "S4GUI out"=w9468:refnum<class "S4GUI.lvclass">)  [unwired: 7 in]
          }
        }
      }
      event "Stop Focus", "Stop Focus 2": Value Change {
        n4022 = event-data() -> ("NewVal"=w9486:bool)  [unwired: 1 in]
        n4023 = case shown="True" w9486 {
          tunnel: w9490 -> [w9492 w9498]
          tunnel: w9489 -> [w9491 w9497]
          tunnel: [w9491 w9496] -> w9488
          tunnel: [w9492 w9495] -> w9487
          frame False {
          }
          frame True {
            n4024 = call-dynamic "Read TelFocus.lvclass.vi"("error in (no error)"=w9497, "S4GUI in"=w9498) -> ("error out"=w9511:errorcluster, "TelFocus.lvclass"=w9512:refnum<class "TelFocus.lvclass">, "S4GUI out"=w9502:refnum<class "S4GUI.lvclass">)  [unwired: 7 in]
            n4025 = call-dynamic "Read SecMirror.lvclass.vi"("error in (no error)"=w9511, "TelFocus in"=w9512) -> ("error out"=w9493:errorcluster, "SecMirror.lvclass"=w9494:refnum<class "SecMirror.lvclass">, "TelFocus out"=w9505:refnum<class "TelFocus.lvclass">)  [unwired: 7 in]
            n4026 = call-dynamic "Read State Machine.vi"("error in (no error)"=w9493, "Device in"=w9494) -> ("error out"=w9509:errorcluster, "State Machine.lvclass"=w9510:refnum<class "State Machine.lvclass">, "Device out"=w9506:refnum<class "SecMirror.lvclass">)  [unwired: 7 in]
            n4027 = call "Next State.vi"("error in (no error)"=w9509, "New_State"=10, "State Machine in"=w9510) -> ("error out"=w9504:errorcluster, "State Machine out"=w9507:refnum<class "State Machine.lvclass">)  [unwired: 7 in]
            n4028 = call-dynamic "Write State Machine.vi"("error in (no error)"=w9504, "State Machine.lvclass"=w9507, "Device in"=w9506) -> ("error out"=w9500:errorcluster, "Device out"=w9499:refnum<class "SecMirror.lvclass">)  [unwired: 7 in]
            n4029 = call-dynamic "Write SecMirror.lvclass.vi"("error in (no error)"=w9500, "SecMirror.lvclass"=w9499, "TelFocus in"=w9505) -> ("error out"=w9501:errorcluster, "TelFocus out"=w9503:refnum<class "TelFocus.lvclass">)  [unwired: 7 in]
            n4030 = call-dynamic "Write TelFocus.lvclass.vi"("error in (no error)"=w9501, "TelFocus.lvclass"=w9503, "S4GUI in"=w9502) -> ("error out"=w9496:errorcluster, "S4GUI out"=w9495:refnum<class "S4GUI.lvclass">)  [unwired: 7 in]
          }
        }
      }
      event "Cooler 1": Value Change {
        n4031 = event-data() -> ("NewVal"=w9545:bool)  [unwired: 1 in]
        n4032 = case shown="False" w9545 {
          tunnel: [w9549 w9551] -> w9521
          tunnel: ["OFF " "ON "] -> w9516
          frame False {
            w9549 = i16 0 items=["Cooler OFF", "Cooler ON"] ("Cooler ON/OFF")
          }
          frame True {
            w9551 = i16 1 items=["Cooler OFF", "Cooler ON"] ("Cooler ON/OFF")
          }
        }
        n4033 = Concatenate Strings("SET COOLER " ("User Event"), w9516, "CLICKED - CH1" ("User Event")) -> (w9514:string)
        n4034 = call-dynamic "Write User Event.vi"("error in (no error)"=w9518, "User Event"=w9514, "S4GUI in"=w9520) -> ("error out"=w9515:errorcluster, "S4GUI out"=w9519:refnum<class "S4GUI.lvclass">)  [unwired: 7 in]
        n4035 = call-dynamic "Read AcquisitionA.vi"("error in (no error)"=w9515, "S4ACS_GUI in"=w9519) -> ("error out"=w9543:errorcluster, "Acquisition.lvclass"=w9544:refnum<class "Acquisition.lvclass">, "S4ACS_GUI out"=w9534:refnum<class "S4GUI.lvclass">)  [unwired: 7 in]
        n4036 = call-dynamic "Read Channel.vi"("error in (no error)"=w9543, "Acquisition in"=w9544) -> ("error out"=w9527:errorcluster, "Channel.lvclass"=w9531:refnum<class "Channel.lvclass">, "Acquisition out"=w9537:refnum<class "Acquisition.lvclass">)  [unwired: 7 in]
        n4037 = call-dynamic "Read Interface.vi"("error in (no error)"=w9527, "Channel in"=w9531) -> ("error out"=w9522:errorcluster, "Interface.lvclass"=w9523:refnum<class "Interface.lvclass">, "Channel out"=w9530:refnum<class "Channel.lvclass">)  [unwired: 7 in]
        n4038 = call-dynamic "Write Cooler ON_OFF.vi"("error in (no error)"=w9522, "Cooler ON/OFF"=w9521, "Interface in"=w9523) -> ("error out"=w9526:errorcluster, "Interface out"=w9528:refnum<class "Interface.lvclass">)  [unwired: 7 in]
        n4039 = call-dynamic "Write Interface.vi"("error in (no error)"=w9526, "Interface.lvclass"=w9528, "Channel in"=w9530) -> ("error out"=w9525:errorcluster, "Channel out"=w9529:refnum<class "Channel.lvclass">)  [unwired: 7 in]
        n4040 = call-dynamic "Read State Machine.vi"("error in (no error)"=w9525, "Device in"=w9529) -> ("error out"=w9541:errorcluster, "State Machine.lvclass"=w9542:refnum<class "State Machine.lvclass">, "Device out"=w9538:refnum<class "Channel.lvclass">)  [unwired: 7 in]
        n4041 = call "Next State.vi"("error in (no error)"=w9541, "New_State"=u32 30, "State Machine in"=w9542) -> ("error out"=w9536:errorcluster, "State Machine out"=w9539:refnum<class "State Machine.lvclass">)  [unwired: 7 in]
        n4042 = call-dynamic "Write State Machine.vi"("error in (no error)"=w9536, "State Machine.lvclass"=w9539, "Device in"=w9538) -> ("error out"=w9532:errorcluster, "Device out"=w9524:refnum<class "Channel.lvclass">)  [unwired: 7 in]
        n4043 = call-dynamic "Write Channel.vi"("error in (no error)"=w9532, "Channel.lvclass"=w9524, "Acquisition in"=w9537) -> ("error out"=w9533:errorcluster, "Acquisition out"=w9535:refnum<class "Acquisition.lvclass">)  [unwired: 7 in]
        n4044 = call-dynamic "Write AcquisitionA.vi"("error in (no error)"=w9533, "Acquisition.lvclass"=w9535, "S4ACS_GUI in"=w9534) -> ("error out"=w9547:errorcluster, "S4ACS_GUI out"=w9546:refnum<class "S4GUI.lvclass">)  [unwired: 7 in]
      }
      event "Cooler 2": Value Change {
        n4045 = event-data() -> ("NewVal"=w9562:bool)  [unwired: 1 in]
        n4046 = case shown="True" w9562 {
          tunnel: [w9588 w9590] -> w9570
          tunnel: ["OFF " ("User Event") "ON " ("User Event")] -> w9556
          frame False {
            w9588 = i16 0 items=["Cooler OFF", "Cooler ON"] ("Cooler ON/OFF")
          }
          frame True {
            w9590 = i16 1 items=["Cooler OFF", "Cooler ON"] ("Cooler ON/OFF")
          }
        }
        n4047 = Concatenate Strings("SET COOLER " ("User Event"), w9556, "CLICKED - CH2" ("User Event")) -> (w9558:string)
        n4048 = call-dynamic "Write User Event.vi"("error in (no error)"=w9554, "User Event"=w9558, "S4GUI in"=w9555) -> ("error out"=w9552:errorcluster, "S4GUI out"=w9553:refnum<class "S4GUI.lvclass">)  [unwired: 7 in]
        n4049 = call "Read AcquisitionB.vi"("error in (no error)"=w9552, "S4ACS_GUI in"=w9553) -> ("error out"=w9567:errorcluster, "Acquisition.lvclass"=w9568:refnum<class "Acquisition.lvclass">, "S4ACS_GUI out"=w9569:refnum<class "S4GUI.lvclass">)  [unwired: 7 in]
        n4050 = call-dynamic "Read Channel.vi"("error in (no error)"=w9567, "Acquisition in"=w9568) -> ("error out"=w9572:errorcluster, "Channel.lvclass"=w9576:refnum<class "Channel.lvclass">, "Acquisition out"=w9579:refnum<class "Acquisition.lvclass">)  [unwired: 7 in]
        n4051 = call-dynamic "Read Interface.vi"("error in (no error)"=w9572, "Channel in"=w9576) -> ("error out"=w9561:errorcluster, "Interface.lvclass"=w9560:refnum<class "Interface.lvclass">, "Channel out"=w9575:refnum<class "Channel.lvclass">)  [unwired: 7 in]
        n4052 = call-dynamic "Write Cooler ON_OFF.vi"("error in (no error)"=w9561, "Cooler ON/OFF"=w9570, "Interface in"=w9560) -> ("error out"=w9571:errorcluster, "Interface out"=w9573:refnum<class "Interface.lvclass">)  [unwired: 7 in]
        n4053 = call-dynamic "Write Interface.vi"("error in (no error)"=w9571, "Interface.lvclass"=w9573, "Channel in"=w9575) -> ("error out"=w9563:errorcluster, "Channel out"=w9574:refnum<class "Channel.lvclass">)  [unwired: 7 in]
        n4054 = call-dynamic "Read State Machine.vi"("error in (no error)"=w9563, "Device in"=w9574) -> ("error out"=w9583:errorcluster, "State Machine.lvclass"=w9584:refnum<class "State Machine.lvclass">, "Device out"=w9580:refnum<class "Channel.lvclass">)  [unwired: 7 in]
        n4055 = call "Next State.vi"("error in (no error)"=w9583, "New_State"=u32 30, "State Machine in"=w9584) -> ("error out"=w9578:errorcluster, "State Machine out"=w9581:refnum<class "State Machine.lvclass">)  [unwired: 7 in]
        n4056 = call-dynamic "Write State Machine.vi"("error in (no error)"=w9578, "State Machine.lvclass"=w9581, "Device in"=w9580) -> ("error out"=w9577:errorcluster, "Device out"=w9564:refnum<class "Channel.lvclass">)  [unwired: 7 in]
        n4057 = call-dynamic "Write Channel.vi"("error in (no error)"=w9577, "Channel.lvclass"=w9564, "Acquisition in"=w9579) -> ("error out"=w9565:errorcluster, "Acquisition out"=w9566:refnum<class "Acquisition.lvclass">)  [unwired: 7 in]
        n4058 = call "Write AcquisitionB.vi"("error in (no error)"=w9565, "Acquisition.lvclass"=w9566, "S4ACS_GUI in"=w9569) -> ("error out"=w9585:errorcluster, "S4ACS_GUI out"=w9586:refnum<class "S4GUI.lvclass">)  [unwired: 7 in]
      }
      event "Cooler 3": Value Change {
        n4059 = event-data() -> ("NewVal"=w9599:bool)  [unwired: 1 in]
        n4060 = case shown="True" w9599 {
          tunnel: [w9627 w9629] -> w9607
          tunnel: ["OFF " "ON "] -> w9595
          frame False {
            w9627 = i16 0 items=["Cooler OFF", "Cooler ON"] ("Cooler ON/OFF")
          }
          frame True {
            w9629 = i16 1 items=["Cooler OFF", "Cooler ON"] ("Cooler ON/OFF")
          }
        }
        n4061 = Concatenate Strings("SET COOLER " ("User Event"), w9595, "CLICKED - CH3" ("User Event")) -> (w9597:string)
        n4062 = call-dynamic "Write User Event.vi"("error in (no error)"=w9593, "User Event"=w9597, "S4GUI in"=w9594) -> ("error out"=w9591:errorcluster, "S4GUI out"=w9592:refnum<class "S4GUI.lvclass">)  [unwired: 7 in]
        n4063 = call-dynamic "Read AcquisitionC.vi"("error in (no error)"=w9591, "S4ACS_GUI in"=w9592) -> ("error out"=w9604:errorcluster, "Acquisition.lvclass"=w9605:refnum<class "Acquisition.lvclass">, "S4ACS_GUI out"=w9606:refnum<class "S4GUI.lvclass">)  [unwired: 7 in]
        n4064 = call-dynamic "Read Channel.vi"("error in (no error)"=w9604, "Acquisition in"=w9605) -> ("error out"=w9610:errorcluster, "Channel.lvclass"=w9615:refnum<class "Channel.lvclass">, "Acquisition out"=w9618:refnum<class "Acquisition.lvclass">)  [unwired: 7 in]
        n4065 = call-dynamic "Read Interface.vi"("error in (no error)"=w9610, "Channel in"=w9615) -> ("error out"=w9609:errorcluster, "Interface.lvclass"=w9612:refnum<class "Interface.lvclass">, "Channel out"=w9614:refnum<class "Channel.lvclass">)  [unwired: 7 in]
        n4066 = call-dynamic "Write Cooler ON_OFF.vi"("error in (no error)"=w9609, "Cooler ON/OFF"=w9607, "Interface in"=w9612) -> ("error out"=w9608:errorcluster, "Interface out"=w9611:refnum<class "Interface.lvclass">)  [unwired: 7 in]
        n4067 = call-dynamic "Write Interface.vi"("error in (no error)"=w9608, "Interface.lvclass"=w9611, "Channel in"=w9614) -> ("error out"=w9600:errorcluster, "Channel out"=w9613:refnum<class "Channel.lvclass">)  [unwired: 7 in]
        n4068 = call-dynamic "Read State Machine.vi"("error in (no error)"=w9600, "Device in"=w9613) -> ("error out"=w9622:errorcluster, "State Machine.lvclass"=w9623:refnum<class "State Machine.lvclass">, "Device out"=w9619:refnum<class "Channel.lvclass">)  [unwired: 7 in]
        n4069 = call "Next State.vi"("error in (no error)"=w9622, "New_State"=u32 30, "State Machine in"=w9623) -> ("error out"=w9617:errorcluster, "State Machine out"=w9620:refnum<class "State Machine.lvclass">)  [unwired: 7 in]
        n4070 = call-dynamic "Write State Machine.vi"("error in (no error)"=w9617, "State Machine.lvclass"=w9620, "Device in"=w9619) -> ("error out"=w9616:errorcluster, "Device out"=w9601:refnum<class "Channel.lvclass">)  [unwired: 7 in]
        n4071 = call-dynamic "Write Channel.vi"("error in (no error)"=w9616, "Channel.lvclass"=w9601, "Acquisition in"=w9618) -> ("error out"=w9602:errorcluster, "Acquisition out"=w9603:refnum<class "Acquisition.lvclass">)  [unwired: 7 in]
        n4072 = call-dynamic "Write AcquisitionC.vi"("error in (no error)"=w9602, "Acquisition.lvclass"=w9603, "S4ACS_GUI in"=w9606) -> ("error out"=w9624:errorcluster, "S4ACS_GUI out"=w9625:refnum<class "S4GUI.lvclass">)  [unwired: 7 in]
      }
      event "Cooler 4": Value Change {
        n4073 = event-data() -> ("NewVal"=w9638:bool)  [unwired: 1 in]
        n4074 = case shown="False" w9638 {
          tunnel: [w9666 w9668] -> w9646
          tunnel: ["OFF" "ON "] -> w9632
          frame False {
            w9666 = i16 0 items=["Cooler OFF", "Cooler ON"] ("Cooler ON/OFF")
          }
          frame True {
